vi "GetTextValue__slk_msxml.vi"(0 "document in":refnum<class "msxml document.lvclass">, 5 "node in":refnum<class "msxml node.lvclass">, 11 "error in (no error)":errorcluster) -> (4 "document out":refnum<class "msxml document.lvclass">, 6 "node out":refnum<class "msxml node.lvclass">, 10 "text value":string, 15 "error out":errorcluster)   [LabVIEW 2020, in "MSXML.lvlib" / "msxml node.lvclass"]
doc: "Returns the text value of MSXML Node."
uses:
  msxml node.lvclass
  MSXML Document/msxml document.lvclass
  msxml node.lvclass/msxml node.ctl
panel:
  # "GetTextValue__slk_msxml.vi\n\nReturns the text value of MSXML Node.\n\nNOTICE -- YOU MUST LEAVE THIS NOTICE IN PLACE.\n\nCopyright (c) 2004-2010 Shawn Liu <shawn.liu.cn@gmail.com>\n\nAll rights reserved."
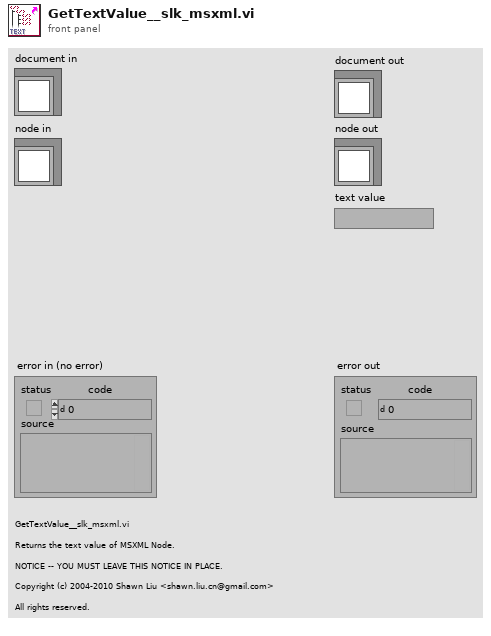
[diagram p1: front panel]
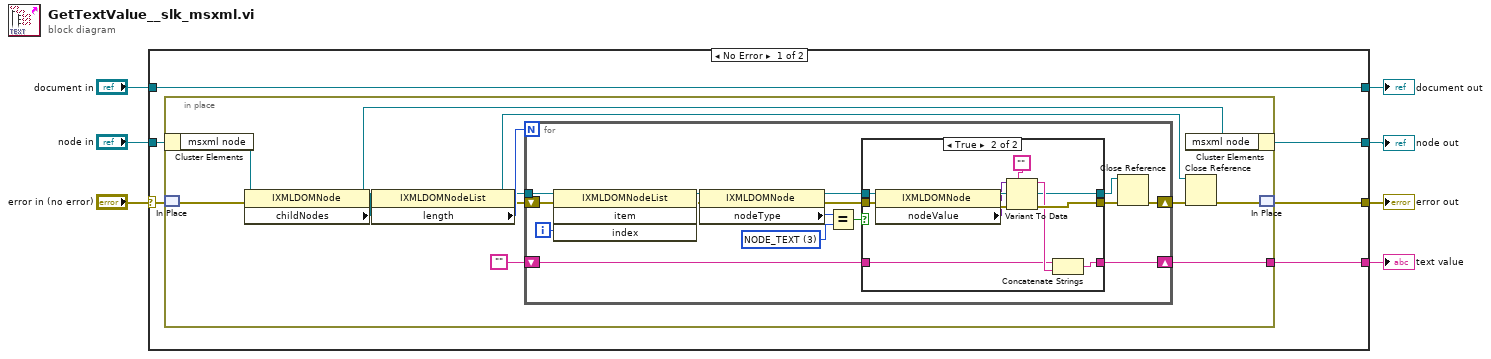
[diagram p0: block diagram]
diagram:
  n1 = case shown="No Error" "error in (no error)" {
    selector: "error in (no error)" -> [w11 w56]
    tunnel: [w10 w56] -> w6
    tunnel: [w13 _] -> w5
    tunnel: "node in" -> [w12 w55]
    tunnel: [w9 w55] -> w3
    tunnel: "document in" -> [w8 w54]
    tunnel: [w8 w54] -> w1
    frame No Error {
      n2 = in-place {
        in-place-border: [w18] -> w13
        n3 = in-place-cluster #1(w12) -> ("msxml node"=w16:refnum<k7>)
        n4 = in-place-match #2(w11) -> (w17:errorcluster)
        n5 = property class="IXMLDOMNode"(reference=w16, error in=w17) -> (reference out=w15:refnum<k7>, error out=w24:errorcluster, "childNodes"=w25:refnum<k7>)
        n6 = property class="IXMLDOMNodeList"(reference=w25, error in=w24) -> (reference out=w19:refnum<k7>, error out=w22:errorcluster, "length"=w23:i32)
        n7 = for {
          N: w23 -> [_]
          shift-right: [w27] -> w20
          shift-left: w22 -> [w39]
          tunnel: w19 -> [w40]
          shift-right: [w29] -> w18
          shift-left: "" -> [w30]
          i -> [w38]
          w34 = 3 items=["NODE_INVALID", "NODE_ELEMENT", "NODE_ATTRIBUTE", "NODE_TEXT", "NODE_CDATA_SECTION", "NODE_ENTITY_REFERENCE", "NODE_ENTITY", "NODE_PROCESSING_INSTRUCTION", "NODE_COMMENT", "NODE_DOCUMENT", "NODE_DOCUMENT_TYPE", "NODE_DOCUMENT_FRAGMENT", "NODE_NOTATION"] ("nodeType")
          n8 = invoke class="IXMLDOMNodeList" method="item"(reference=w40, error in=w39, "index"=w38) -> (error out=w36:errorcluster, "item"=w37:refnum<k7>)  [unwired: 1 in, 2 out]
          n9 = property class="IXMLDOMNode"(reference=w37, error in=w36) -> (reference out=w31:refnum<k7>, error out=w32:errorcluster, "nodeType"=w35:i32)
          n10 = Equal?(x=w35, y=w34) -> (x = y?=w33:bool)
          n11 = case shown="True" w33 {
            tunnel: [w43 w51] -> w28
            tunnel: [w41 w50] -> w29
            tunnel: [w42 w48] -> w26
            tunnel: w32 -> [w43 w47]
            tunnel: w31 -> [w42 w46]
            tunnel: w30 -> [w41 w45]
            frame False {
            }
            frame True {
              n12 = property class="IXMLDOMNode"(reference=w46, error in=w47) -> (reference out=w48:refnum<k7>, error out=w53:errorcluster, "nodeValue"=w44:variant)
              n13 = Variant To Data(error in=w53, type="", Variant=w44) -> (data=w49:string, error out=w51:errorcluster)
              n14 = Concatenate Strings(w45, w49) -> (w50:string)
            }
          }
          n15 = Close Reference(reference=w26, error in (no error)=w28) -> (error out=w27:errorcluster)
        }
        n16 = in-place-cluster #1("msxml node"=w15) -> (w9:refnum<class "msxml node.lvclass">)
        n17 = Close Reference(reference=w19, error in (no error)=w20) -> (error out=w14:errorcluster)
        n18 = in-place-match #2(w14) -> (w10:errorcluster)
      }
    }
    frame Error {
    }
  }
  "node out" <- w3
  "error out" <- w6
  "text value" <- w5
  "document out" <- w1
